vi "Dummy.vi"   [LabVIEW 2025, in "jettl.lvlib"]
uses:
  jettl.lvlib
  jettl Tools/_Template/Templates/TEMPLATE Actor/TEMPLATE Actor.lvlib
  Transport/Transport/Transport.lvclass
  Core Actor/Core Actor.lvlib
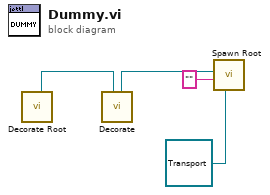
[diagram p0: block diagram]
diagram:
  n1 = call "Decorate Root.vi"() -> ("Actor out"=w1:refnum<class "Actor.lvclass">)  [unwired: 11 in]
  n2 = call "Decorate.vi"("Actor"=w1) -> ("Decorated Actor"=w4:refnum<class "Actor.lvclass">)  [unwired: 10 in]
  n3 = call "Spawn Root.vi"("Transport"=refnum<class "Transport.lvclass"> refnum, "UID"="", "Actor"=w4) -> ()  [unwired: 7 in, 2 out]
